vi "setreinitMicroscope.vi"(0 "Microscope in":refnum<class "Microscope.lvclass">, 1 "microscope event queue":refnum<queue>, 2 "image event queue":refnum<queue>, 3 "error in (no error)":errorcluster, 4 "acquire?":bool) -> (5 "Microscope out":refnum<class "Microscope.lvclass">, 7 "error out":errorcluster)   [LabVIEW 2012, in "Microscope.lvclass"]
uses:
  classes/Microscope.lvclass
  typedefs/MicroscopeEvent.ctl
  typedefs/ImageEvent.ctl
  classes/Microscope.lvclass/Microscope.ctl
  sequences/partial_stop_sequence.vi
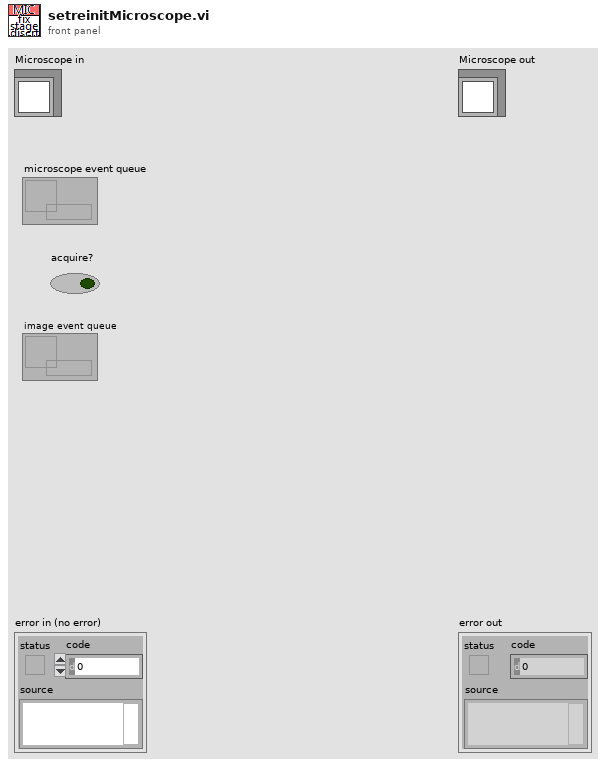
[diagram p1: front panel]
types:
  T1 = typedef "Scan Type.ctl" = enum16{"None", "Point", "Full Image Continuous", "Full Image Grab"}
  T2 = typedef "DetectorType.ctl" = enum16{"PMT", "SpectraWiz"}
  T3 = typedef "Move Type.ctl" = enum16{"None", "Continuous", "Discrete"}
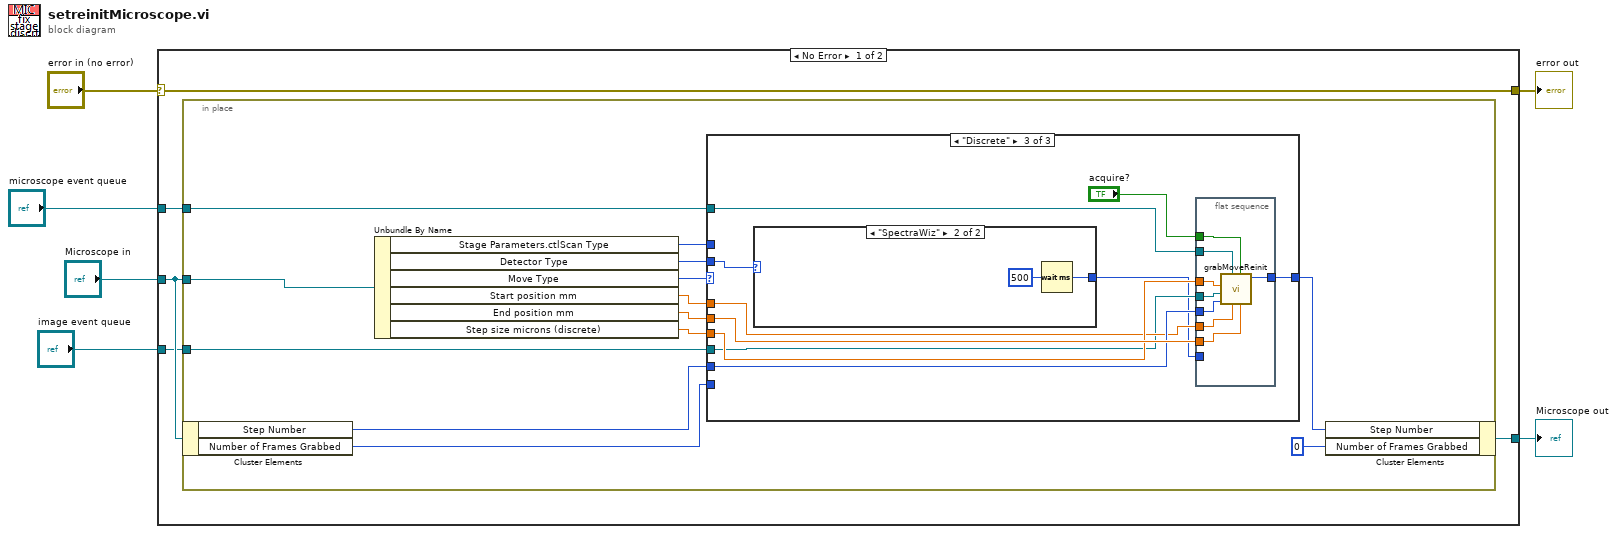
[diagram p0: block diagram]
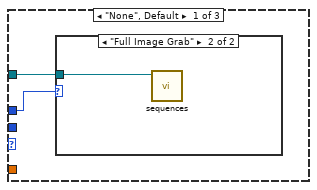
[diagram p2: hidden frame]
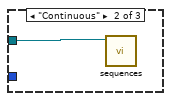
[diagram p4: hidden frame]
diagram:
  n1 = case shown="No Error" "error in (no error)" {
    selector: "error in (no error)" -> [w11 w50]
    tunnel: [w11 w50] -> w5
    tunnel: [w8 w49] -> w3
    tunnel: "Microscope in" -> [w9 w49]
    tunnel: "microscope event queue" -> [w10 _]
    tunnel: "image event queue" -> [w7 _]
    frame No Error {
      n2 = in-place {
        in-place-border: w9 -> [w24]
        in-place-border: w10 -> [w22]
        in-place-border: w7 -> [w14]
        n3 = in-place-cluster #1(w9) -> ("Step Number"=w18:i32, "Number of Frames Grabbed"=w16:i32)
        n4 = Unbundle By Name(w24) -> ("Stage Parameters.ctlScan Type"=w12:T1, "Detector Type"=w13:T2, "Move Type"=w23:T3, "Start position mm"=w21:dbl, "End position mm"=w20:dbl, "Step size microns (discrete)"=w19:dbl)
        n5 = case shown="\"Discrete\"" w23 {
          tunnel: w22 -> [w26 w28 w37]
          tunnel: w21 -> [_ _ w34]
          tunnel: w20 -> [_ _ w38]
          tunnel: w19 -> [_ _ w35]
          tunnel: w18 -> [_ _ w36]
          tunnel: [_ _ w33] -> w17
          tunnel: w16 -> [_ _ _]
          tunnel: w14 -> [_ _ w32]
          tunnel: w13 -> [_ _ w30]
          tunnel: w12 -> [w25 _ _]
          frame "None", Default {
            n6 = case shown="\"Full Image Grab\"" w25 {
              tunnel: w26 -> [_ w27]
              frame "None", Default {
              }
              frame "Full Image Grab" {
                n7 = call-poly "sequences.vi"("Queue in"=w27) -> ()  [unwired: 9 in, 2 out]
              }
            }
          }
          frame "Continuous" {
            n8 = call-poly "sequences.vi"("Queue in"=w28) -> ()  [unwired: 9 in, 2 out]
          }
          frame "Discrete" {
            n9 = case shown="\"SpectraWiz\"" w30 {
              tunnel: [_ w40] -> w31
              frame "PMT", Default {
              }
              frame "SpectraWiz" {
                n10 = Wait (ms)(milliseconds to wait=u32 500) -> (millisecond timer value=w40:u32)
              }
            }
            n11 = flat-sequence {
              tunnel: w38 -> [w48]
              tunnel: w37 -> [w47]
              tunnel: w34 -> [w44]
              tunnel: [w43] -> w33
              tunnel: "acquire?" -> [w41]
              tunnel: w36 -> [w46]
              tunnel: w35 -> [w45]
              tunnel: w32 -> [w42]
              tunnel: w31 -> [_]
              frame #0 {
                n12 = call "grabMoveReinit.vi"("End position mm"=w48, "acquire?"=w41, "Start position mm"=w44, "microscope event queue"=w47, "Step Number in"=w46, "image event queue"=w42, "Step size microns (discrete)"=w45) -> ("Step Number out"=w43:i32)  [unwired: 4 in]
              }
            }
          }
        }
        n13 = in-place-cluster #1("Step Number"=w17, "Number of Frames Grabbed"=0) -> (w8:refnum<class "Microscope.lvclass">)
      }
    }
    frame Error {
    }
  }
  "error out" <- w5
  "Microscope out" <- w3
